vi "GetStates.vi"(0 "Pump_1AI_1DO_2DI in":refnum<class "PM_Group.lvclass">, 11 "error in":errorcluster) -> (6 "PMG":T1, 15 "error out":errorcluster)   [LabVIEW 2019, in "PM_Group.lvclass"]
uses:
  PM_Group.lvclass
  TypeDef/State PMG.ctl
  TypeDef/PMG Mode.ctl
  TypeDef/State Engine 2.ctl
  TypeDef/State Engine.ctl
  PM_Group.lvclass/PM_Group.ctl
  Device_class/Device.lvclass/Device.ctl
  Engine_1DO_2DI_class/Engine_1DO_2DI.lvclass/Engine_1DO_2DI.ctl
  Device_class/GetFPGA.vi
  Engine_1DO_2DI_class/Engine_1DO_2DI.lvclass
  C:/Users/ANENKOV_V1/Desktop/src/Device_class/Device.lvclass
  FPGA_API_class/FPGA API.lvclass
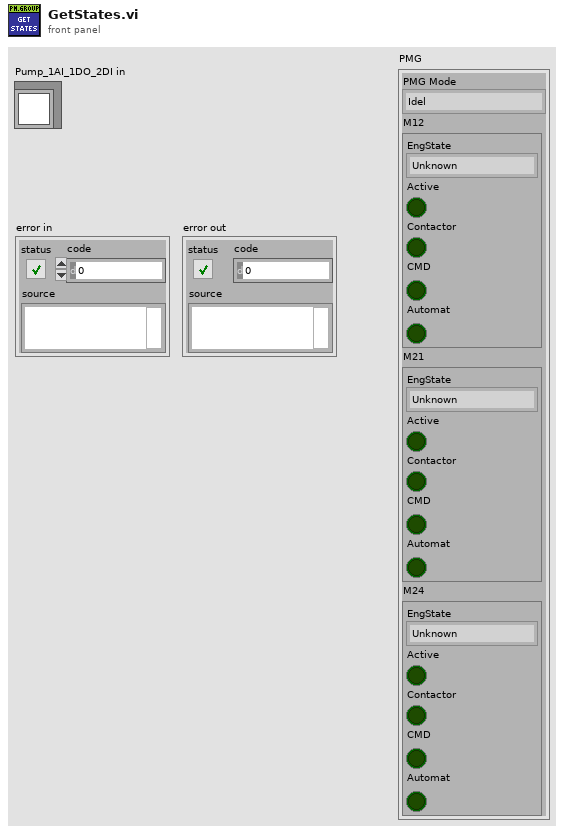
[diagram p1: front panel]
types:
  T1 = typedef "State PMG.ctl" = cluster{"PMG Mode":T2, "M12":T3, "M21":T3, "M24":T3}
  T2 = typedef "PMG Mode.ctl" = enum16{"Idel", "Filling", "Pressure"}
  T3 = typedef "State Engine 2.ctl" = cluster{"EngState":T4, "Active":bool, "Contactor":bool, "CMD":bool, "Automat":bool}
  T4 = typedef "State Engine.ctl" = enum16{"Unknown", "Off", "TupningOn", "On", "TurningOff"}
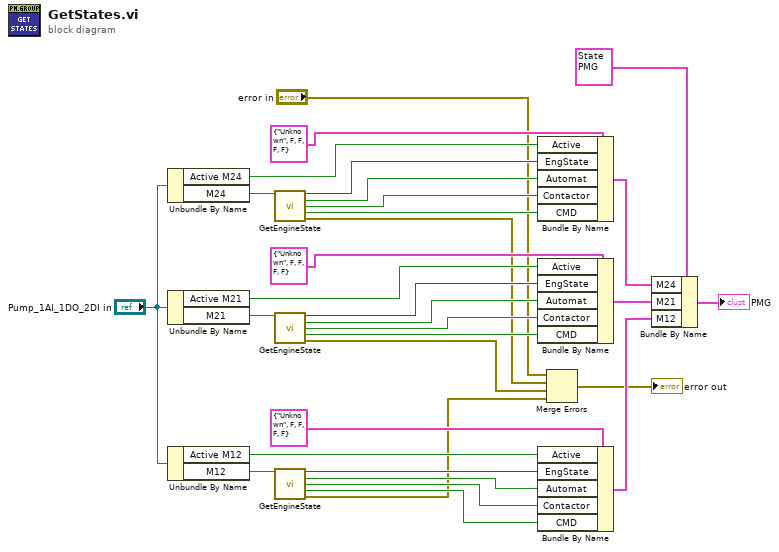
[diagram p0: block diagram]
diagram:
  n1 = Unbundle By Name("Pump_1AI_1DO_2DI in") -> ("Active M24"=w25:bool, "M24"=w32:refnum<class "Engine_1DO_2DI.lvclass">)
  n2 = Unbundle By Name("Pump_1AI_1DO_2DI in") -> ("Active M21"=w11:bool, "M21"=w17:refnum<class "Engine_1DO_2DI.lvclass">)
  n3 = Unbundle By Name("Pump_1AI_1DO_2DI in") -> ("Active M12"=w24:bool, "M12"=w18:refnum<class "Engine_1DO_2DI.lvclass">)
  n4 = call "GetEngineState.vi"("Engine"=w32) -> ("EngineState"=w29:T4, "Automat"=w28:bool, "Contactor"=w27:bool, "DO Cmd"=w26:bool, "error out"=w3:errorcluster)  [unwired: 10 in]
  n5 = call "GetEngineState.vi"("Engine"=w17) -> ("EngineState"=w15:T4, "Automat"=w14:bool, "Contactor"=w13:bool, "DO Cmd"=w12:bool, "error out"=w4:errorcluster)  [unwired: 10 in]
  n6 = call "GetEngineState.vi"("Engine"=w18) -> ("EngineState"=w20:T4, "Automat"=w21:bool, "Contactor"=w22:bool, "DO Cmd"=w23:bool, "error out"=w5:errorcluster)  [unwired: 10 in]
  n7 = Bundle By Name(cluster=T3 {"EngState"=enum."Unknown", "Active"=FALSE, "Contactor"=FALSE, "CMD"=FALSE, "Automat"=FALSE} ("M12"), "Active"=w25, "EngState"=w29, "Automat"=w28, "Contactor"=w27, "CMD"=w26) -> (w8:T3)
  n8 = Bundle By Name(cluster=T3 {"EngState"=enum."Unknown", "Active"=FALSE, "Contactor"=FALSE, "CMD"=FALSE, "Automat"=FALSE} ("M12"), "Active"=w11, "EngState"=w15, "Automat"=w14, "Contactor"=w13, "CMD"=w12) -> (w7:T3)
  n9 = Bundle By Name(cluster=T3 {"EngState"=enum."Unknown", "Active"=FALSE, "Contactor"=FALSE, "CMD"=FALSE, "Automat"=FALSE} ("M12"), "Active"=w24, "EngState"=w20, "Automat"=w21, "Contactor"=w22, "CMD"=w23) -> (w6:T3)
  n10 = Merge Errors("error in", w3, w4, w5) -> (→"error out":errorcluster)
  n11 = Bundle By Name(cluster=T1 {"PMG Mode"=enum."Idel", "M12"={"EngState"=enum."Unknown", "Active"=FALSE, "Contactor"=FALSE, "CMD"=FALSE, "Automat"=FALSE}, "M21"={"EngState"=enum."Unknown", "Active"=FALSE, "Contactor"=FALSE, "CMD"=FALSE, "Automat"=FALSE}, "M24"={"EngState"=enum."Unknown", "Active"=FALSE, "Contactor"=FALSE, "CMD"=FALSE, "Automat"=FALSE}} ("PMG"), "M24"=w8, "M21"=w7, "M12"=w6) -> (→"PMG":T1)
